vi "Update 433x Info.vi"(8 "error in (no error)":errorcluster) -> (0 "error IO":errorcluster, 3 "Board Info for checking":T1)   [LabVIEW 2011, in "PXIe-433x Custom Device.lvlib"]
uses:
  PXIe-433x Custom Device.lvlib
  Board Info for checking settings.ctl
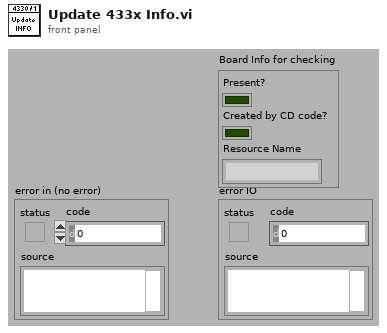
[diagram p1: front panel]
types:
  T1 = typedef "PXIe-433x Custom Device.lvlib/Board Info for checking settings.ctl" = cluster{"Present?":bool, "Created by CD code?":bool, "Resource Name":string}
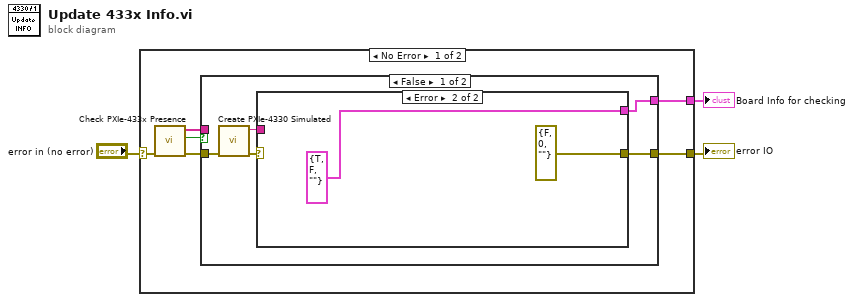
[diagram p0: block diagram]
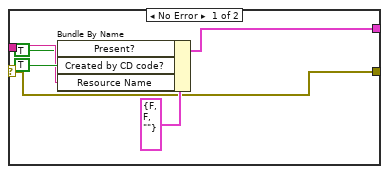
[diagram p2: hidden frame]
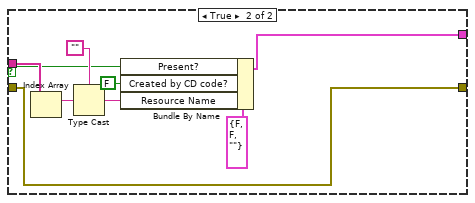
[diagram p3: hidden frame]
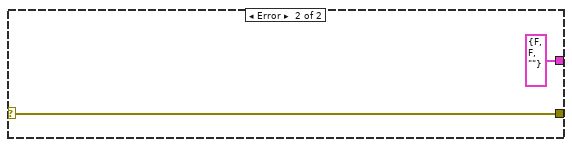
[diagram p4: hidden frame]
diagram:
  n1 = case shown="No Error" "error in (no error)" {
    selector: "error in (no error)" -> [w8 w33]
    tunnel: [w9 w33] -> w2
    tunnel: [w7 T1 {"Present?"=FALSE, "Created by CD code?"=FALSE, "Resource Name"=""} ("Board Info for checking")] -> w1
    frame No Error {
      n2 = call "Check PXIe-433x Presence.vi"("error in (no error)"=w8) -> ("error out"=w5:errorcluster, "PXIe-433x Present?"=w6:bool, "PXIe-433x Resources"=w4:tag[])  [unwired: 8 in]
      n3 = case shown="False" w6 {
        selector: w6 -> [_ w23]
        tunnel: w5 -> [w14 w25]
        tunnel: w4 -> [_ w28]
        tunnel: [w11 w25] -> w9
        tunnel: [w10 w24] -> w7
        frame False {
          n4 = call "Create PXIe-4330 Simulated.vi"("error in (no error)"=w14) -> ("error out"=w13:errorcluster, "Actual Dev Name"=w12:string)  [unwired: 9 in]
          n5 = case shown="Error" w13 {
            selector: w13 -> [w17 _]
            tunnel: w12 -> [w18 _]
            tunnel: [w17 errorcluster {"status"=FALSE, "code"=0, "source"=""} ("error IO")] -> w11
            tunnel: [w15 T1 {"Present?"=TRUE, "Created by CD code?"=FALSE, "Resource Name"=""} ("Board Info for checking")] -> w10
            frame No Error {
              n6 = Bundle By Name(cluster=T1 {"Present?"=FALSE, "Created by CD code?"=FALSE, "Resource Name"=""} ("Board Info for checking"), "Present?"=TRUE, "Created by CD code?"=TRUE, "Resource Name"=w18) -> (w15:T1)
            }
            frame Error {
            }
          }
        }
        frame True {
          n7 = Index Array(array=w28) -> (element=w27:tag)  [unwired: 1 in]
          n8 = Type Cast(type="", x=w27) -> (*(type *) &x=w26:string)
          n9 = Bundle By Name(cluster=T1 {"Present?"=FALSE, "Created by CD code?"=FALSE, "Resource Name"=""} ("Board Info for checking"), "Present?"=w23, "Created by CD code?"=FALSE, "Resource Name"=w26) -> (w24:T1)
        }
      }
    }
    frame Error {
    }
  }
  "error IO" <- w2
  "Board Info for checking" <- w1
